vi "Graph to GraphViz String.vi"(11 "Abstract Graph":refnum<class "Abstract Graph.lvclass">) -> (3 "Graphviz String":string)   [LabVIEW 2021, in "GraphLib.lvlib" / "Abstract Graph.lvclass"]
uses:
  Abstract Graph.lvclass
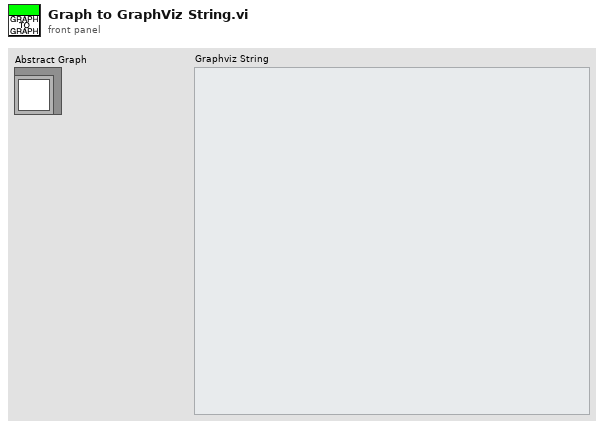
[diagram p1: front panel]
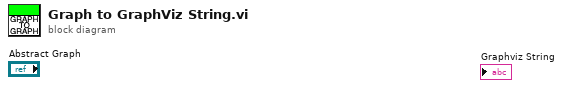
[diagram p0: block diagram]
diagram:
